vi "Demo.vi"() -> ()   [LabVIEW 2020]
uses:
  function01.ctl
  function02.ctl
  function03.ctl
  function04.ctl
  function05.ctl
  function06.ctl
  function07.ctl
  <vilib>/measure/NI_MABase.lvlib
panel:
  in  "Select":T1(radio)
  out "Graph":waveform(dbl)(graph)
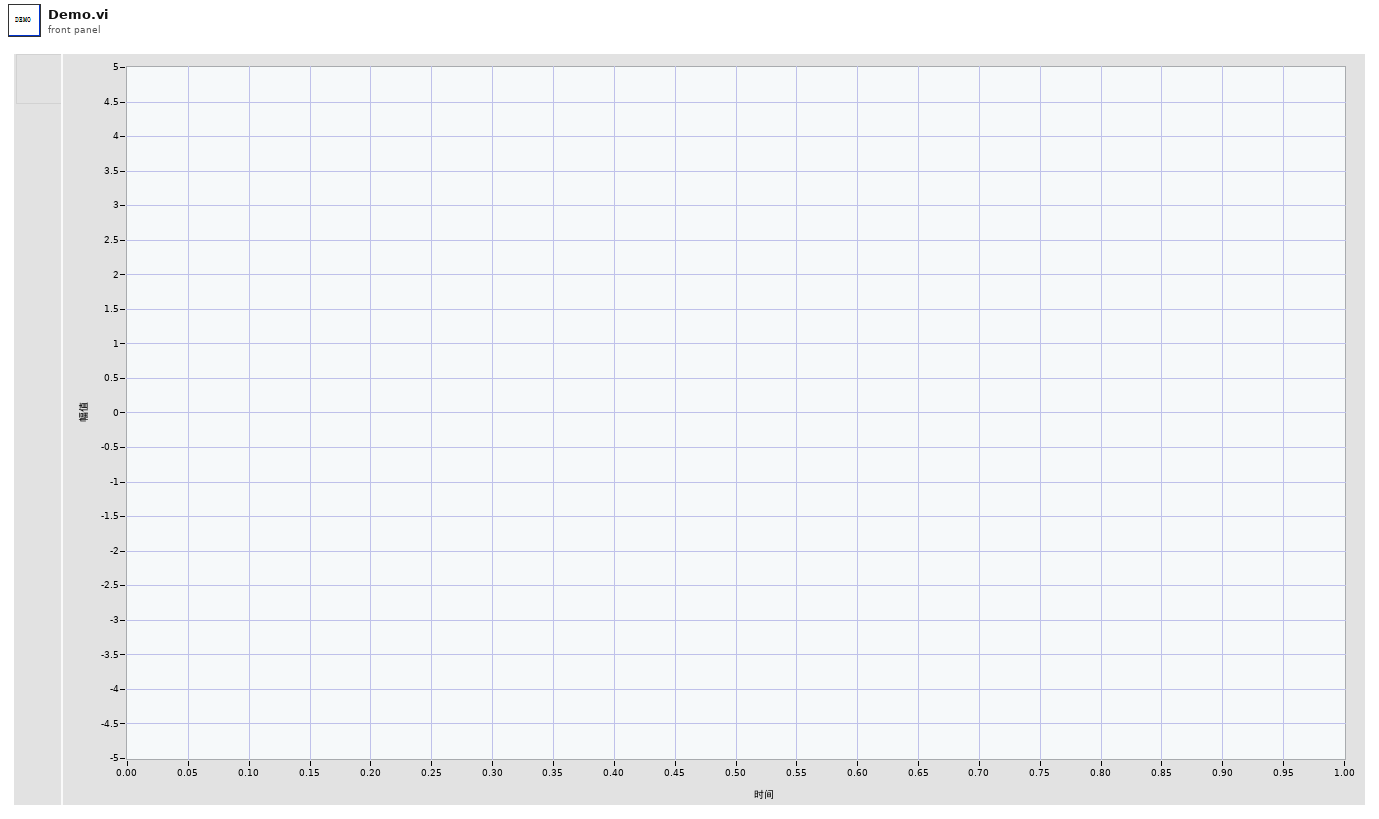
[diagram p1: front panel]
types:
  T1 = enum32{"单选选项1", "单选选项2", "单选选项2 2", "单选选项2 3", "单选选项2 4", "单选选项2 5", "单选选项2 6"}
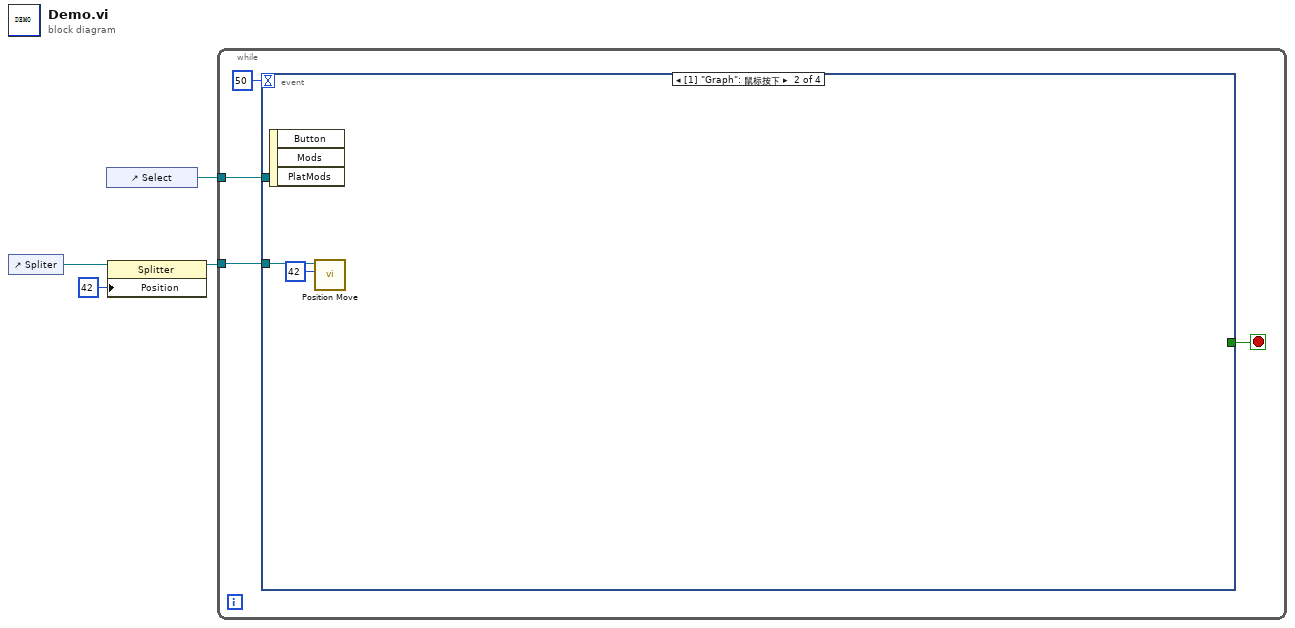
[diagram p0: block diagram]
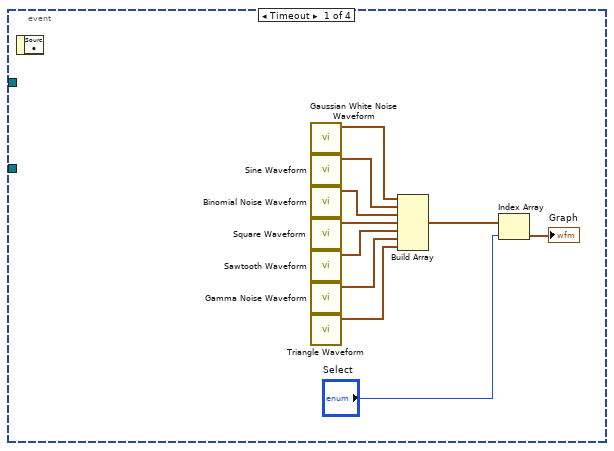
[diagram p2: hidden frame]
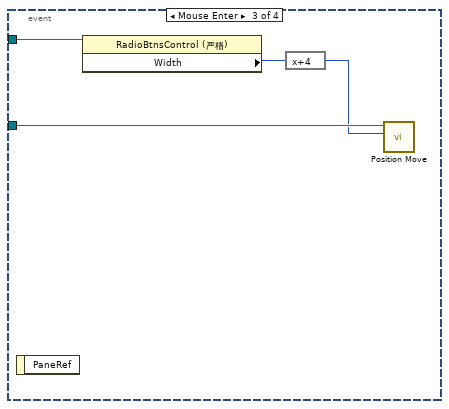
[diagram p3: hidden frame]
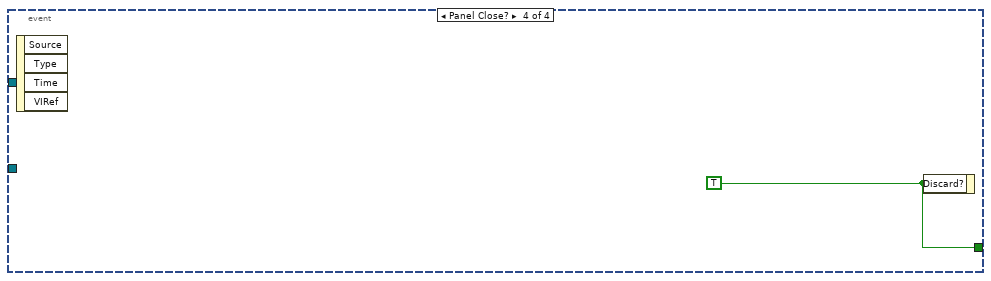
[diagram p4: hidden frame]
diagram:
  n1 = control-ref of="Spliter"() -> (w1:refnum<vi>)
  n2 = control-ref of="Select"() -> (w3:refnum<vi>)
  n3 = property class="Splitter"(reference=w1, "Position"=42 ("分隔栏位置")) -> (reference out=w2:refnum<vi>)  [unwired: 1 in, 1 out]
  n4 = while {
    tunnel: w2 -> [w7]
    tunnel: w3 -> [w6]
    stop <- w8 stop-if-true
    n5 = event shown="[1] \"Graph\": 鼠标按下" {
      selector: _ -> [_ _ _ _]
      dyn-events: _ -> [_ _ _ _]
      timeout: 50 -> [_ _ _ _]
      tunnel: [_ _ _ w25] -> w8
      tunnel: w7 -> [_ w20 w24 _]
      tunnel: w6 -> [_ _ w23 _]
      event Timeout {
        n6 = event-data() -> ()  [unwired: 1 in, 1 out]
        n7 = call <vilib>:"Gaussian White Noise Waveform.vi"() -> ("signal out"=w13:waveform(dbl))  [unwired: 10 in, 1 out]
        n8 = call <vilib>:"Sine Waveform.vi"() -> ("signal out"=w14:waveform(dbl))  [unwired: 10 in, 1 out]
        n9 = call <vilib>:"Binomial Noise Waveform.vi"() -> ("signal out"=w15:waveform(u32))  [unwired: 10 in, 1 out]
        n10 = call <vilib>:"Square Waveform.vi"() -> ("signal out"=w16:waveform(dbl))  [unwired: 10 in, 1 out]
        n11 = call <vilib>:"Sawtooth Waveform.vi"() -> ("signal out"=w17:waveform(dbl))  [unwired: 10 in, 1 out]
        n12 = call <vilib>:"Gamma Noise Waveform.vi"() -> ("signal out"=w18:waveform(dbl))  [unwired: 10 in, 1 out]
        n13 = call <vilib>:"Triangle Waveform.vi"() -> ("signal out"=w10:waveform(dbl))  [unwired: 10 in, 1 out]
        n14 = Build Array(w13, w14, w15, w16, w17, w18, w10) -> (w12:waveform(dbl)[])
        n15 = Index Array(array=w12, index="Select") -> (element=→"Graph":waveform(dbl))
      }
      event "Graph": Mouse Down {
        n16 = event-data() -> ()  [unwired: 1 in, 3 out]
        n17 = call "Position Move.vi"("Target"=42 ("分隔栏位置"), "分隔栏"=w20) -> ()  [unwired: 10 in]
      }
      event Mouse Enter {
        n18 = event-data() -> ()  [unwired: 1 in, 1 out]
        n19 = property class="RadioBtnsControl (严格)"(reference=w23) -> ("Width"=w22:u32)  [unwired: 1 in, 2 out]
        n20 = expression code="x+4"(w22) -> (w21:u32)
        n21 = call "Position Move.vi"("Target"=w21, "分隔栏"=w24) -> ()  [unwired: 10 in]
      }
      event Panel Close? {
        w25 = TRUE ("放弃？")
        n22 = event-data() -> ()  [unwired: 1 in, 4 out]
        n23 = event-data("Discard?"=w25) -> ()  [unwired: 1 in, 1 out]
      }
    }
  }
